vi "3_VisualAD_Report(Dataset).vi"() -> ()   [LabVIEW 2020]
uses:
  <vilib>/Ngene/DeepLTK Anomaly Detection Addon/DeepLTK_Anomaly_Detection_Addon/API/Controls/Feature_Scorer_Params.ctl
  <vilib>/Ngene/DeepLTK Anomaly Detection Addon/DeepLTK_Anomaly_Detection_Addon/API/Controls/Gaussian_Blur.ctl
  <vilib>/Ngene/DeepLTK Anomaly Detection Addon/DeepLTK_Anomaly_Detection_Addon/API/Controls/NN_Paths.ctl
  subVIs/Visualizer/Controls/Display_Options.ctl
  subVIs/Visualizer/Controls/ROI_Display_Options.ctl
  subVIs/Visualizer/Controls/Heatmap_Display_Options.ctl
  subVIs/Visualizer/Controls/ColorMap.ctl
  <vilib>/Ngene/DeepLTK Anomaly Detection Addon/DeepLTK_Anomaly_Detection_Addon/API/Controls/MinMax.ctl
  <vilib>/Ngene/DeepLTK Anomaly Detection Addon/DeepLTK_Anomaly_Detection_Addon/API/Controls/NNPC_Setup.ctl
  <vilib>/Ngene/Deep Learning Toolkit/Toolkit/NN_Data/API/NN_Dims(C,H,W).ctl
  <vilib>/Ngene/Deep Learning Toolkit/Toolkit/NN_Network/Controls/NN_Device.ctl
  <vilib>/Analysis/baseanly.llb/Mean (DBL).vi
  <vilib>/Ngene/DeepLTK Anomaly Detection Addon/DeepLTK_Anomaly_Detection_Addon/API/NNPC_Predict/NNPC_Predict(Single).vi
  <vilib>/Ngene/DeepLTK Anomaly Detection Addon/DeepLTK_Anomaly_Detection_Addon/DeepLTK_Anomaly_Detection_Addon.lvlib
  <vilib>/Analysis/NI_AALBase.lvlib
  <vilib>/Ngene/Deep Learning Toolkit/Toolkit/Deep_Learning_Toolkit_by_Ngene.lvlib
panel:
  in  "NNPC_Setup":T1={"Input_Dims"={"C"=-1, "H"=-1, "W"=-1}, "mBatch"=1, "Device"=enum."GPU", "GPU Id"=0}
  in  "Display_Options":T4={"ROI_Options"={"Color"=16860, "Width"=3, "Drawing Mode"=enum."Frame"}, "Heatmap_Options"={"ColorMap"=enum."Jet", "Alpha"=0.4, "Heatmap_Range"={"Min"=-1.0, "Max"=-1.0}}, "Has GT?"=FALSE} {"Heatmap_Options"."Heatmap_Range"."Min" format="%#_5g"}
  in  "NNPC_Paths":T9={"CFG"=path "D:/Ngene/GitHub/deepltk_examples/3_Image_Processing/36_Anomaly_Detection/Models/NNPC_Cards_3ofHearts__25_03_28__20_34_36/NNPC_Cards_3ofHearts.cfg", "BIN"=path "D:/Ngene/GitHub/deepltk_examples/3_Image_Processing/36_Anomaly_Detection/Models/NNPC_Cards_3ofHearts__25_03_28__20_34_36/NNPC_Cards_3ofHearts.bin"}
  out "Detection Results":T10(plugin-control)
  out "dt_Predict":dbl=0.006085650000095484 format="%#_4p"
  in  "Feature_Scorer_Params":T11={"Nearest_Neighbors"=1, "Calculate Anomaly Map"=TRUE, "Gaussian_Blur"={"Kernel_Size"=33, "Sigma"=4.0}}
  out "Actual_Pixel_Threshold":sgl=10.0
  out "Total":i32=50
  out "Progress":i32=49
  in  "Dest. Path":path=path "D:/Results"
  out "dT_ImRead":dbl=0.002772512000010465 format="%#_4p"
  in  "Ground_Truth_Folder_Path":path
  in  "Pixel_Thrshld(Custom)":sgl=10.0 format="%_5g"
  in  "Image_Dataset_Folder_Path":path=path "D:/Ngene/GitHub/deepltk_examples/3_Image_Processing/36_Anomaly_Detection/Dataset/Playing_Cards_3ofHearts/test"
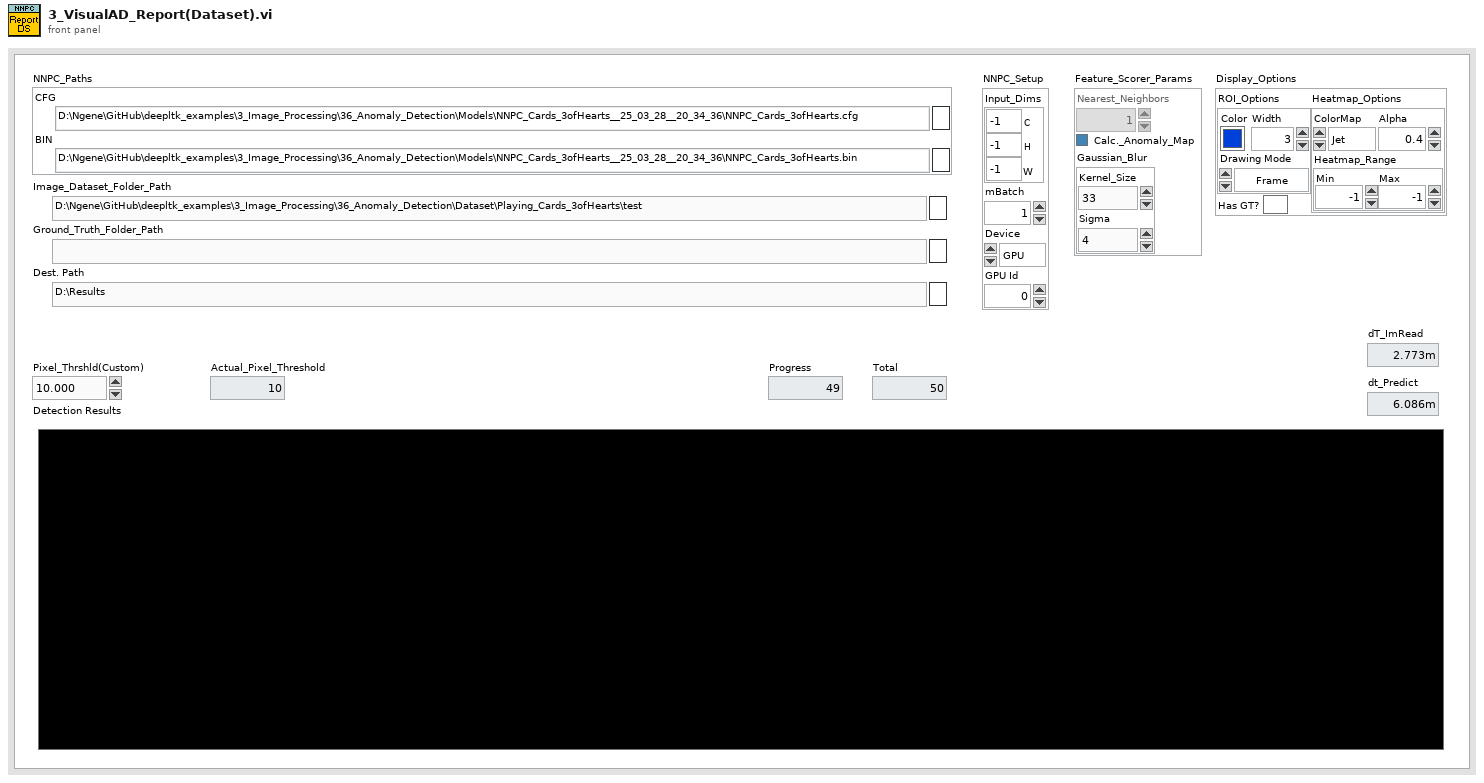
[diagram p1: front panel]
types:
  T1 = typedef "DeepLTK_Anomaly_Detection_Addon.lvlib/NNPC_Setup.ctl" = cluster{"Input_Dims":T2, "mBatch":i32, "Device":T3, "GPU Id":i32}
  T2 = typedef "Deep_Learning_Toolkit_by_Ngene.lvlib/NN_Dims(C,H,W).ctl" = cluster{"C":i32, "H":i32, "W":i32}
  T3 = typedef "Deep_Learning_Toolkit_by_Ngene.lvlib/NN_Device.ctl" = enum16{"CPU", "GPU"}
  T4 = typedef "Display_Options.ctl" = cluster{"ROI_Options":T5, "Heatmap_Options":T6, "Has GT?":bool}
  T5 = typedef "ROI_Display_Options.ctl" = cluster{"Color":u32, "Width":u32, "Drawing Mode":enum16{"Frame", "Fill"}}
  T6 = typedef "Heatmap_Display_Options.ctl" = cluster{"ColorMap":T7, "Alpha":sgl, "Heatmap_Range":T8}
  T7 = typedef "ColorMap.ctl" = enum16{"Jet", "Perula", "Inferno", "Plasma", "Viridis"}
  T8 = typedef "DeepLTK_Anomaly_Detection_Addon.lvlib/MinMax.ctl" = cluster{"Min":sgl, "Max":sgl}
  T9 = typedef "DeepLTK_Anomaly_Detection_Addon.lvlib/NN_Paths.ctl" = cluster{"CFG":path, "BIN":path}
  T10 = typedef "IMAQ Image.ctl" = refnum<image>
  T11 = typedef "DeepLTK_Anomaly_Detection_Addon.lvlib/Feature_Scorer_Params.ctl" = cluster{"Nearest_Neighbors":i32, "Calculate Anomaly Map":bool, "Gaussian_Blur":T12}
  T12 = typedef "DeepLTK_Anomaly_Detection_Addon.lvlib/Gaussian_Blur.ctl" = cluster{"Kernel_Size":i32, "Sigma":sgl}
  T13 = typedef "DeepLTK_Anomaly_Detection_Addon.lvlib/NNPC_Evaluation_Results.ctl" = cluster{"Threshold(Image)":sgl, "Threshold(Pixel)":sgl, "Pixel_Range":cluster{"Min":sgl, "Max":sgl}}
  T14 = typedef "DeepLTK_Anomaly_Detection_Addon.lvlib/NNPC_PreProcessing_Options.ctl" = cluster{"DS_Name":string, "Input_Dims":T2, "Center Crop Size":i32, "Interpolation Type":u32, "Dataset_Stats":T15}
  T15 = typedef "DeepLTK_Anomaly_Detection_Addon.lvlib/NNPC_DS_Stats.ctl" = cluster{"means":T16, "stds":T16}
  T16 = typedef "DeepLTK_Anomaly_Detection_Addon.lvlib/Image_Stats_RGB.ctl" = cluster{"R":sgl, "G":sgl, "B":sgl}
  T17 = typedef "DeepLTK_Anomaly_Detection_Addon.lvlib/NNPC_Instance.ctl" = cluster{"NN":T18, "MemBank_Data":T33, "Name":string}
  T18 = typedef "Deep_Learning_Toolkit_by_Ngene.lvlib/NN.ctl" = cluster{"Name":string, "No of Layers":i32, "mBatch":i32, "Layers":T19[], "Dimty":T20, "Dims_In":T2, "Dims_Out":T2, "Working_Dir":path, "Train?":bool, "Train_Params":T21, "LR_Update_Policy":T24, "Session Data":T26, "Ground_truth":T27, "NNg_hdls":T28, "NN_Device":T3, "GPU Id":i32, "Labels":string[], "Receptive Field":T29[], "Loss_Type":T30, "Loss_Cfg_Prms":variant, "NNG_WS":T31}
  T19 = typedef "Deep_Learning_Toolkit_by_Ngene.lvlib/NN_Layer_ref.ctl" = refnum<data-value>
  T20 = typedef "Deep_Learning_Toolkit_by_Ngene.lvlib/NN_In_Out_Dim-ty.ctl" = enum8{"In1D_Out1D", "In3D_Out1D", "In3D_Out3D", "In3D_OutBBox"}
  T21 = typedef "Deep_Learning_Toolkit_by_Ngene.lvlib/NN_Train_Params.ctl" = cluster{"Optimizer":T22, "Beta_1":sgl, "Beta_2":sgl, "Weight Decay(L1)":sgl, "Weight Decay(L2)":sgl, "Data_Sampling":T23}
  T22 = typedef "Deep_Learning_Toolkit_by_Ngene.lvlib/NN_Train_Optimizer.ctl" = enum16{"SGD", "Adam", "Adagrad", "Adadelta", "RMSProp", "Nesterov"}
  T23 = typedef "Deep_Learning_Toolkit_by_Ngene.lvlib/NN_Train_Data_Sampling.ctl" = enum16{"Random", "Sequential"}
  T24 = typedef "Deep_Learning_Toolkit_by_Ngene.lvlib/NN_LR_Policy_Cfg.ctl" = cluster{"Policy_Type":T25, "LR0":dbl, "k":sgl, "WarmUp_Policy":enum16{"Step", "Ramp"}, "WarmUp_Iter":i32, "WarmUp_Ratio":sgl}
  T25 = typedef "Deep_Learning_Toolkit_by_Ngene.lvlib/NN_LR_Policy_Type.ctl" = enum16{"Manual", "Step", "Exp", "1/t"}
  T26 = typedef "Deep_Learning_Toolkit_by_Ngene.lvlib/NN_Train_Session_Data.ctl" = cluster{"Epochs":sgl, "Tot_Iter":i32, "LR":sgl, "LR_iter":i32}
  T27 = typedef "Deep_Learning_Toolkit_by_Ngene.lvlib/NN_Ground_truth.ctl" = cluster{"Y":variant}
  T28 = typedef "Deep_Learning_Toolkit_by_Ngene.lvlib/nng_cuda_handles.ctl" = cluster{"cudnn":u64, "cublas":u64, "stream":u64, "curand":u64}
  T29 = typedef "Deep_Learning_Toolkit_by_Ngene.lvlib/NN_Dims(V,H).ctl" = cluster{"V":i32, "H":i32}
  T30 = typedef "Deep_Learning_Toolkit_by_Ngene.lvlib/NN_Loss_Type.ctl" = enum16{"None", "MSE", "CrossEntropy", "YOLO_v2", "YOLO_v4"}
  T31 = typedef "Deep_Learning_Toolkit_by_Ngene.lvlib/NNG_WS.ctl" = cluster{"NNG_WS_Mem":T32, "Max_WS_Size":i64}
  T32 = typedef "Deep_Learning_Toolkit_by_Ngene.lvlib/NNg_WS_Mem_DVR.ctl" = refnum<data-value>
  T33 = typedef "DeepLTK_Anomaly_Detection_Addon.lvlib/MemBank_and_Norm_Variants.ctl" = cluster{"MemBank":variant, "MemBank Norm":variant}
  T34 = typedef "Anomaly_Detection_Results_Imgs.ctl" = cluster{"Image":T10, "Ground Truth":T10, "Predicted Heat Map":T10, "Predicted Mask":T10, "Segmentation":T10}
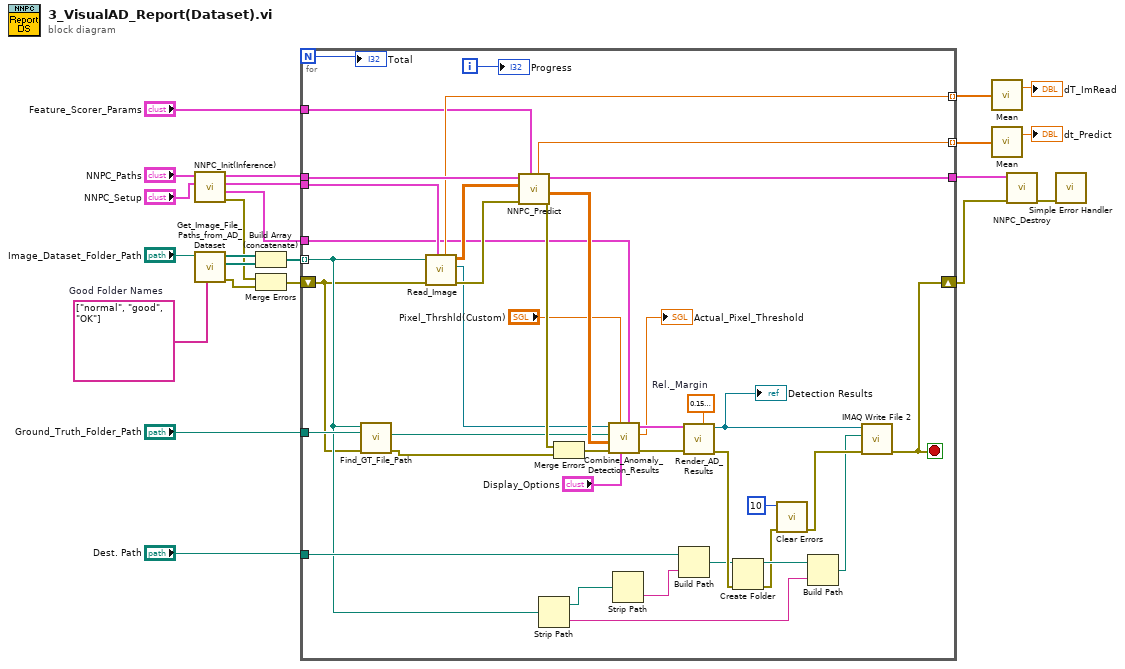
[diagram p0: block diagram]
diagram:
  w1 = string[] ["normal", "good", "OK"]  # Good Folder Names
  n1 = call <vilib>:"NNPC_Init(Inference).vi"("NNPC_Setup"="NNPC_Setup", "NNPC_Paths"="NNPC_Paths") -> ("error out"=w7:errorcluster, "Evaluation_Results"=w3:T13, "PreProc_Options"=w5:T14, "NNPC_out"=w20:T17)  [unwired: 5 in, 1 out]
  n2 = call "Get_Image_File_Paths_from_AD_Dataset.vi"("Good Folder Names"=w1, "Dataset Folder"="Image_Dataset_Folder_Path") -> ("error out"=w19:errorcluster, "Bad Dataset Files"=w13:path[], "Good Dataset Files"=w14:path[])  [unwired: 7 in]
  n3 = Build Array (concatenate)(w14, w13) -> (w12:path[])
  n4 = Merge Errors(w7, w19) -> (w6:errorcluster)
  n5 = for {
    N -> [w44]
    shift-right: [w50] -> w22
    shift-left: w6 -> [w32]
    tunnel: w12 -> [w38] mode=indexing
    tunnel: w20 -> [w56]
    tunnel: [w59] -> w9
    tunnel: [w53] -> w17 mode=indexing
    tunnel: [w40] -> w16 mode=indexing
    tunnel: "Dest. Path" -> [w51]
    tunnel: "Ground_Truth_Folder_Path" -> [w42]
    tunnel: "Feature_Scorer_Params" -> [w35]
    tunnel: w5 -> [w29]
    tunnel: w3 -> [w28]
    i -> [w45]
    stop <- w50 stop-if-true
    w26 = sgl 0.15  # Rel._Margin
    n6 = call "Find_GT_File_Path.vi"("error in"=w32, "GT Mask Folder Path"=w42, "Image File Path"=w38) -> ("error out"=w30:errorcluster, "GT File Path"=w41:path)  [unwired: 5 in, 2 out]
    n7 = call "Read_Image.vi"("PreProcessing_Options"=w29, "error in"=w32, "Img Path"=w38) -> ("error out"=w55:errorcluster, "Imaq Image Out"=w25:T10, "Image Out"=w34:sgl[][][], "dT_Img_Read"=w53:dbl)  [unwired: 5 in]
    n8 = call-poly <vilib>:"NNPC_Predict.vi"("Feature_Scorer_Params"=w35, "error in"=w55, "Image_in"=w34, "NNPC_in"=w56) -> ("error out"=w60:errorcluster, "Anomaly_Map"=w58:sgl[][], "NNPC_out"=w59:T17, "dT_Predict"=w40:dbl)  [unwired: 3 in, 1 out]
    n9 = Strip Path(path=w38) -> (stripped path=w52:path, name=w27:string)
    n10 = Merge Errors(w60, w30) -> (w31:errorcluster)
    n11 = call "Combine_Anomaly_Detection_Results.vi"("Evaluation_Results"=w28, "Display_Options"="Display_Options", "Pixel Anomaly Thrshld"="Pixel_Thrshld(Custom)", "error in"=w31, "Anomaly Map"=w58, "Gt File Path"=w41, "Orig Image In"=w25) -> ("error out"=w33:errorcluster, "Actual Pixel Threshold"=→"Actual_Pixel_Threshold":sgl, "Anomaly Detection Rresults"=w57:T34)  [unwired: 2 in]
    n12 = Strip Path(path=w52) -> (name=w36:string)  [unwired: 1 out]
    n13 = Build Path(base path=w51, name or relative path=w36) -> (appended path=w37:path)
    n14 = call "Render_AD_Results.vi"("Rel._Margin"=w26, "error in"=w33, "Anomaly Detection Rresults"=w57) -> ("error out"=w61:errorcluster, "Anomaly Detection Results"=w39:T10)  [unwired: 7 in]
    "Detection Results" <- w39
    n15 = Create Folder(path (use dialog)=w37, error in=w61) -> (created path=w48:path, error out=w47:errorcluster)  [unwired: 1 in, 1 out]
    n16 = call <vilib>:"Clear Errors.vi"("error in (no error)"=w47, "specific error code to clear (0: all)"=10) -> ("error out"=w62:errorcluster)  [unwired: 4 in, 1 out]
    n17 = Build Path(base path=w48, name or relative path=w27) -> (appended path=w49:path)
    n18 = call-poly "IMAQ Write File 2"("error in (no error)"=w62, "File Path"=w49, "Image"=w39) -> ("error out"=w50:errorcluster)  [unwired: 7 in, 1 out]
    "Progress" <- w45
    "Total" <- w44
  }
  n19 = call-poly <vilib>:"Mean.vi"("X"=w17) -> ("mean"=→"dT_ImRead":dbl)  [unwired: 1 out]
  n20 = call-poly <vilib>:"Mean.vi"("X"=w16) -> ("mean"=→"dt_Predict":dbl)  [unwired: 1 out]
  n21 = call <vilib>:"NNPC_Destroy.vi"("error in"=w22, "NNPC_in"=w9) -> ("error out"=w21:errorcluster)  [unwired: 9 in]
  n22 = call <vilib>:"Simple Error Handler.vi"("error in (no error)"=w21) -> ()  [unwired: 4 in, 5 out]
